vi "CRYSUpper_Lowerness Check.vi"(0 "Limits":u16(ring)=2 items=["Upper Only", "Lower Only", "Upper & Lower"], 4 "Lo unit":string, 5 "Data unit":string, 6 "Up unit":string, 7 "Type":u16, 8 "Lo source":u16, 9 "Up source":u16, 10 "Lower limit":cluster{"Numeric":dbl, "Numeric 2":dbl}[](array[cluster]) {"Numeric 2" format="%.2f"; "Numeric" format="%.2f"}, 11 "Upper limit":cluster{"Numeric":dbl, "Numeric 2":dbl}[](array[cluster]) {"Numeric 2" format="%.2f"; "Numeric" format="%.2f"}) -> (3 "Do save":bool)   [LabVIEW 2013]
uses:
  <vilib>/Analysis/baseanly.llb/Mean (DBL).vi
  <vilib>/Analysis/NI_AALBase.lvlib
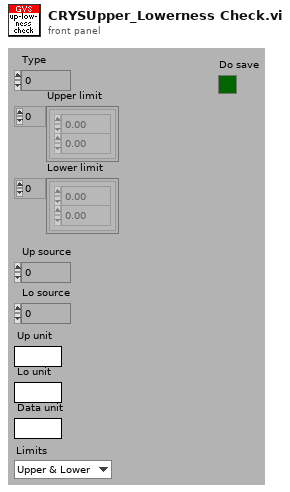
[diagram p1: front panel]
types:
  T1 = enum16{"OK", "Yes", "YesNo", "YesNoCancel", "ReplaceAppend"}
  T2 = enum16{"Left Button", "Center Button", "Right Button", "Window Close"}
  T3 = typedef "CRYData Cluster.ctl" = cluster{"Name":string, "Curve":cluster{"x":dbl, "y":dbl, "z":dbl}[], "X data":u16, "Y data":u16, "Z data":u16, "X axis":u16, "Y axis":u16, "Z axis":u16, "X unit":string, "Y unit":string, "Z unit":string, "X dB ref":dbl, "Y dB ref":dbl, "Z dB ref":dbl, "single val":bool, "protected":bool, "display X":bool, "display Y":bool, "display Z":bool, "Test Info":string, "Step No.":i32, "Plot Settings":cluster{"Color":u32, "Interpolation":u8, "Point Style":u8, "Line Style":u8, "Point Color":u32, "Line Width":u8, "Bar Plot Style":u8, "Fill To":i16}, "AutoProtect":bool}
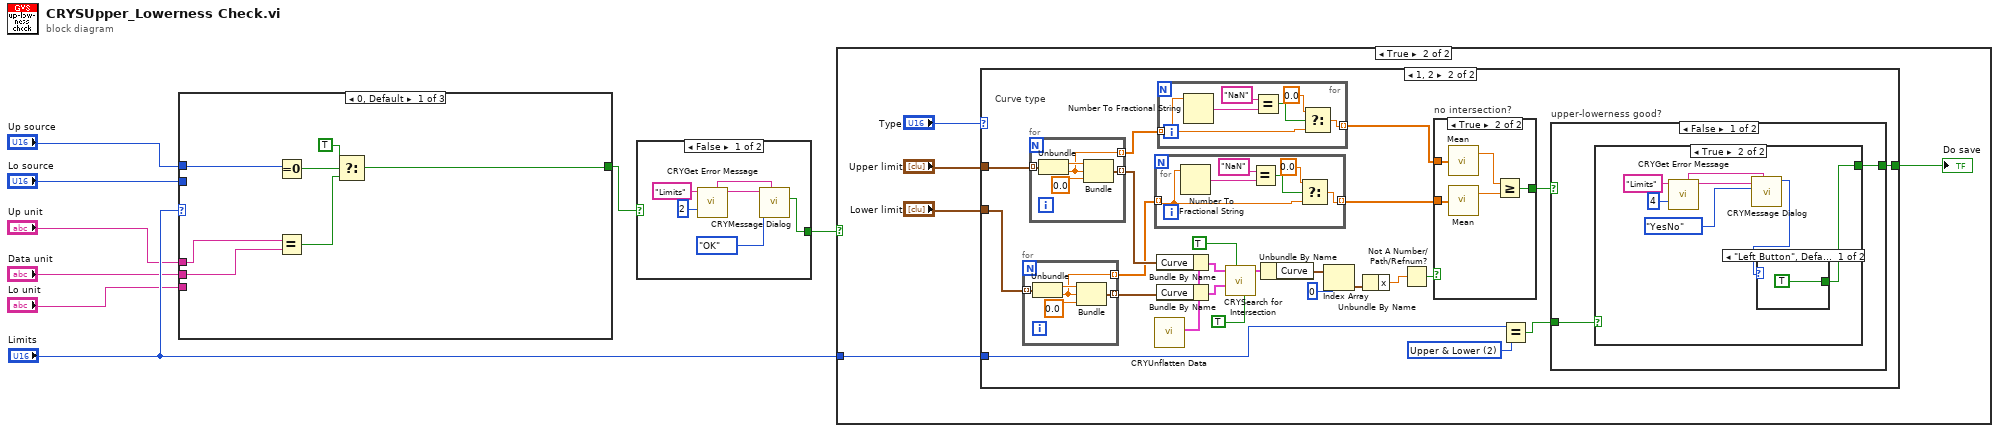
[diagram p0: block diagram]
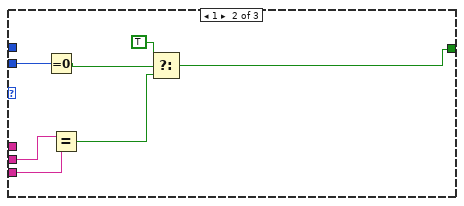
[diagram p2: hidden frame]
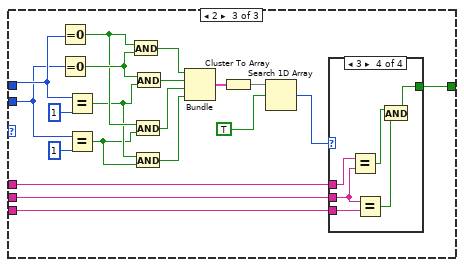
[diagram p3: hidden frame]
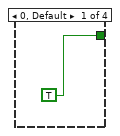
[diagram p4: hidden frame]
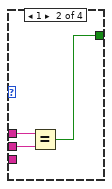
[diagram p5: hidden frame]
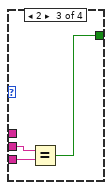
[diagram p6: hidden frame]
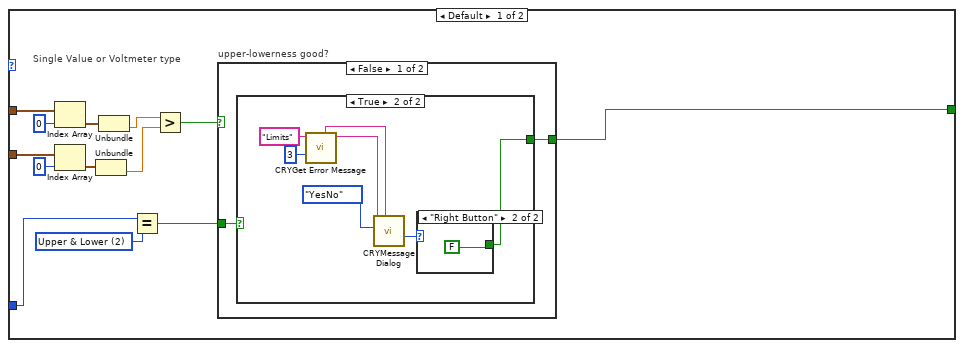
[diagram p9: hidden frame]
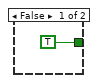
[diagram p10: hidden frame]
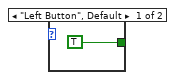
[diagram p11: hidden frame]
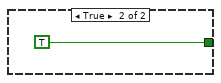
[diagram p12: hidden frame]
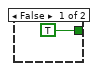
[diagram p13: hidden frame]
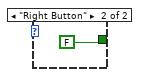
[diagram p14: hidden frame]
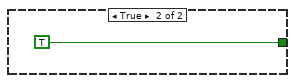
[diagram p15: hidden frame]
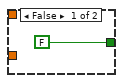
[diagram p16: hidden frame]
diagram:
  n1 = case shown="0, Default" "Limits" {
    tunnel: "Up source" -> [w15 _ w41]
    tunnel: "Up unit" -> [w12 _ w25]
    tunnel: "Data unit" -> [w11 w19 w24]
    tunnel: [w9 w16 w26] -> w1
    tunnel: "Lo source" -> [_ w22 w38]
    tunnel: "Lo unit" -> [_ w18 w23]
    frame 0, Default {
      n2 = Equal To 0?(x=w15) -> (x = 0?=w14:bool)
      n3 = Equal?(x=w12, y=w11) -> (x = y?=w10:bool)
      n4 = Select(t=TRUE, s=w14, f=w10) -> (s? t:f=w9:bool)
    }
    frame 1 {
      n5 = Equal To 0?(x=w22) -> (x = 0?=w20:bool)
      n6 = Equal?(x=w19, y=w18) -> (x = y?=w17:bool)
      n7 = Select(t=TRUE, s=w20, f=w17) -> (s? t:f=w16:bool)
    }
    frame 2 {
      n8 = Equal To 0?(x=w41) -> (x = 0?=w37:bool)
      n9 = Equal To 0?(x=w38) -> (x = 0?=w40:bool)
      n10 = Equal?(x=w41, y=u16 1) -> (x = y?=w36:bool)
      n11 = Equal?(x=w38, y=u16 1) -> (x = y?=w35:bool)
      n12 = And(x=w37, y=w40) -> (x .and. y?=w31:bool)
      n13 = And(x=w37, y=w35) -> (x .and. y?=w29:bool)
      n14 = And(x=w36, y=w35) -> (x .and. y?=w28:bool)
      n15 = And(x=w40, y=w36) -> (x .and. y?=w30:bool)
      n16 = Bundle(w31, w30, w29, w28) -> (w34:cluster{bool, bool, bool, bool})  [unwired: 1 out]
      n17 = Cluster To Array(cluster=w34) -> (array=w32:bool[])
      n18 = Search 1D Array(1D array=w32, element=TRUE) -> (index of element=w27:i32)  [unwired: 1 out]
      n19 = case shown="3" w27 {
        tunnel: [TRUE w44 w47 w50] -> w26
        tunnel: w25 -> [_ w46 _ w55]
        tunnel: w24 -> [_ w45 w49 w54]
        tunnel: w23 -> [_ _ w48 w53]
        frame 0, Default {
        }
        frame 1 {
          n20 = Equal?(x=w46, y=w45) -> (x = y?=w44:bool)
        }
        frame 2 {
          n21 = Equal?(x=w49, y=w48) -> (x = y?=w47:bool)
        }
        frame 3 {
          n22 = Equal?(x=w55, y=w54) -> (x = y?=w52:bool)
          n23 = Equal?(x=w54, y=w53) -> (x = y?=w51:bool)
          n24 = And(x=w52, y=w51) -> (x .and. y?=w50:bool)
        }
      }
    }
  }
  n25 = case shown="False" w1 {
    selector: w1 -> [_ w62]
    tunnel: [w58 w62] -> w8
    frame False {
      n26 = call "CRYGet Error Message.vi"("Error No"=2, "Kind"="Limits") -> ("Message"=w59:string, "Window Title"=w56:string)  [unwired: 4 in, 4 out]
      n27 = call "CRYMessage Dialog.vi"("Window Title"=w56, "YesNoCancel"=T1."OK", "Message Content"=w59) -> ("YesNo"=w58:bool)  [unwired: 7 in, 1 out]
    }
    frame True {
    }
  }
  n28 = case shown="True" w8 {
    tunnel: "Limits" -> [_ w63]
    frame False {
    }
    frame True {
      n29 = case shown="1, 2" "Type" {
        tunnel: "Upper limit" -> [w78 w114]
        tunnel: "Lower limit" -> [w77 w115]
        tunnel: [w79 w112] -> w64
        tunnel: w63 -> [w69 w99]
        frame Default {
          w70 = u16 2 items=["Upper Only", "Lower Only", "Upper & Lower"] ("Limits")
          # "Single Value or Voltmeter type"
          n30 = Index Array(array=w78, index=0) -> (element=w74:cluster{"Numeric":dbl, "Numeric 2":dbl})
          n31 = Index Array(array=w77, index=0) -> (element=w72:cluster{"Numeric":dbl, "Numeric 2":dbl})
          n32 = Unbundle(w72) -> ("Numeric 2"=w71:dbl)  [unwired: 1 out]
          n33 = Unbundle(w74) -> ("Numeric 2"=w73:dbl)  [unwired: 1 out]
          n34 = Equal?(x=w69, y=w70) -> (x = y?=w68:bool)
          n35 = Greater?(x=w73, y=w71) -> (0:w80:bool)
          n36 = case "upper-lowerness good?" shown="False" w80 {
            tunnel: [w82 TRUE] -> w79
            tunnel: w68 -> [w81 _]
            frame False {
              n37 = case shown="True" w81 {
                tunnel: [TRUE w90] -> w82
                frame False {
                }
                frame True {
                  n38 = call "CRYGet Error Message.vi"("Error No"=3, "Kind"="Limits") -> ("Message"=w87:string, "Window Title"=w86:string)  [unwired: 4 in, 4 out]
                  n39 = call "CRYMessage Dialog.vi"("Window Title"=w86, "YesNoCancel"=T1."YesNo", "Message Content"=w87) -> ("Which Button?"=w84:T2)  [unwired: 7 in, 1 out]
                  n40 = case shown="\"Right Button\"" w84 {
                    tunnel: [TRUE FALSE] -> w90
                    frame "Left Button", Default {
                    }
                    frame "Right Button" {
                    }
                  }
                }
              }
            }
            frame True {
            }
          }
        }
        frame 1, 2 {
          w101 = u16 2 items=["Upper Only", "Lower Only", "Upper & Lower"] ("Limits")
          # "Curve type"
          n41 = for {
            tunnel: w115 -> [w153] mode=indexing
            tunnel: [w150] -> w108 mode=indexing
            tunnel: [w149] -> w96 mode=indexing
            n42 = Unbundle(w153) -> ("Numeric"=w152:dbl, "Numeric 2"=w149:dbl)
            n43 = Bundle("Numeric"=w152, "Numeric 2"=w149, 0.0) -> (w150:cluster{"Numeric":dbl, "Numeric 2":dbl, dbl})  [unwired: 1 out]
          }
          n44 = for {
            tunnel: w114 -> [w158] mode=indexing
            tunnel: [w155] -> w109 mode=indexing
            tunnel: [w154] -> w97 mode=indexing
            n45 = Unbundle(w158) -> ("Numeric"=w157:dbl, "Numeric 2"=w154:dbl)
            n46 = Bundle("Numeric"=w157, "Numeric 2"=w154, 0.0) -> (w155:cluster{"Numeric":dbl, "Numeric 2":dbl, dbl})  [unwired: 1 out]
          }
          n47 = for {
            tunnel: w96 -> [w118] mode=indexing
            tunnel: [w119] -> w94 mode=indexing
            n48 = Number To Fractional String(number=w118) -> (F-format string=w120:string)  [unwired: 3 out]
            n49 = Equal?(x="NaN", y=w120) -> (x = y?=w122:bool)
            n50 = Select(t=0.0, s=w122, f=w118) -> (s? t:f=w119:dbl)
          }
          n51 = call "CRYUnflatten Data.vi"() -> ("Datum"=w102:T3)  [unwired: 1 in, 10 out]
          n52 = Bundle By Name(cluster=w102, "Curve"=w109) -> (w107:T3)
          n53 = Bundle By Name(cluster=w102, "Curve"=w108) -> (w98:T3)
          n54 = for {
            tunnel: w97 -> [w126] mode=indexing
            tunnel: [w124] -> w95 mode=indexing
            n55 = Number To Fractional String(number=w126) -> (F-format string=w129:string)  [unwired: 3 out]
            n56 = Equal?(x="NaN", y=w129) -> (x = y?=w127:bool)
            n57 = Select(t=0.0, s=w127, f=w126) -> (s? t:f=w124:dbl)
          }
          n58 = call "CRYSearch for Intersection.vi"("All points"=TRUE, "Supress warnings (F)"=TRUE, "Operand B"=w98, "Operand A"=w107) -> ("Resulting data"=w106:T3)  [unwired: 2 in, 5 out]
          n59 = Unbundle By Name(w106) -> ("Curve"=w103:cluster{"x":dbl, "y":dbl, "z":dbl}[])
          n60 = Index Array(array=w103, index=0 ("Index")) -> (element=w111:cluster{"x":dbl, "y":dbl, "z":dbl})
          n61 = Unbundle By Name(w111) -> ("x"=w110:dbl)
          n62 = Not A Number/Path/Refnum?(number/path/refnum=w110) -> (NaN/Path/Refnum?=w116:bool)
          n63 = case "no intersection?" shown="True" w116 {
            tunnel: w95 -> [_ w148]
            tunnel: w94 -> [_ w147]
            tunnel: [FALSE w144] -> w113
            frame False {
            }
            frame True {
              n64 = call-poly <vilib>:"Mean.vi"("X"=w148) -> ("mean"=w145:dbl)  [unwired: 1 out]
              n65 = call-poly <vilib>:"Mean.vi"("X"=w147) -> ("mean"=w146:dbl)  [unwired: 1 out]
              n66 = Greater Or Equal?(x=w145, y=w146) -> (x >= y?=w144:bool)
            }
          }
          n67 = Equal?(x=w99, y=w101) -> (x = y?=w100:bool)
          n68 = case "upper-lowerness good?" shown="False" w113 {
            tunnel: [w131 TRUE] -> w112
            tunnel: w100 -> [w130 _]
            frame False {
              n69 = case shown="True" w130 {
                tunnel: [TRUE w139] -> w131
                frame False {
                }
                frame True {
                  n70 = call "CRYGet Error Message.vi"("Error No"=4, "Kind"="Limits") -> ("Message"=w136:string, "Window Title"=w135:string)  [unwired: 4 in, 4 out]
                  n71 = call "CRYMessage Dialog.vi"("Window Title"=w135, "YesNoCancel"=T1."YesNo", "Message Content"=w136) -> ("Which Button?"=w133:T2)  [unwired: 7 in, 1 out]
                  n72 = case shown="\"Left Button\", Default" w133 {
                    tunnel: [TRUE FALSE] -> w139
                    frame "Left Button", Default {
                    }
                    frame "Right Button" {
                    }
                  }
                }
              }
            }
            frame True {
            }
          }
        }
      }
      "Do save" <- w64
    }
  }
